vi "ma_Process DC for 1 Block.vi"(6 "reset":bool, 7 "window for DC":T2(ring)=enum."Hanning", 8 "time signal data (samples)":dbl[](array[numeric])=[1.0, 1.0] format="%0.2p", 10 "averaging type":enum16{"Linear", "Exponential"}(ring), 11 "state info":T1 {"buffer" format="%0.2f"; "timestamp" format="%<%.4X>T"; "dt history" format="%0.2f"; "t0 history" format="%<%I:%M:%S%4u %p>T"; "exp TC (samples)" format="%0.2f"; "RMS history" format="%0.2f"; "DC history" format="%0.2f"}) -> (2 "DC value data":dbl=-262128.0 format="%0.6p", 3 "state info":T1 {"buffer" format="%0.2f"; "timestamp" format="%<%.4X>T"; "dt history" format="%0.2f"; "t0 history" format="%<%I:%M:%S%4u %p>T"; "exp TC (samples)" format="%0.2f"; "RMS history" format="%0.2f"; "DC history" format="%0.2f"})   [LabVIEW 2020, in "NI_MAPro.lvlib"]
uses:
  NI_MAPro.lvlib
  NI_AALBase.lvlib
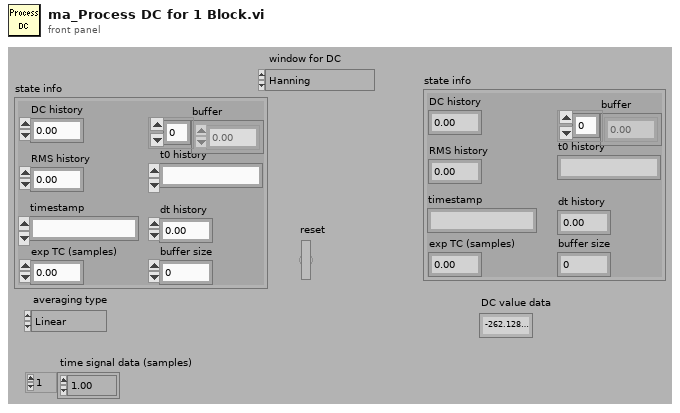
[diagram p1: front panel]
types:
  T1 = cluster{"DC history":dbl, "RMS history":dbl, "exp TC (samples)":dbl, "buffer size":i32, "t0 history":timestamp, "dt history":dbl, "timestamp":timestamp, "buffer":dbl[]}
  T2 = enum16{"Rectangular (none)", "Hanning", "Low side lobe"}
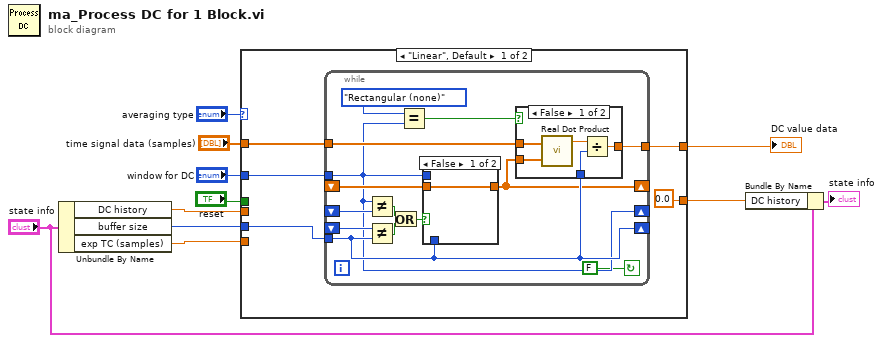
[diagram p0: block diagram]
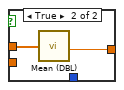
[diagram p2: hidden frame]
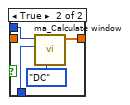
[diagram p3: hidden frame]
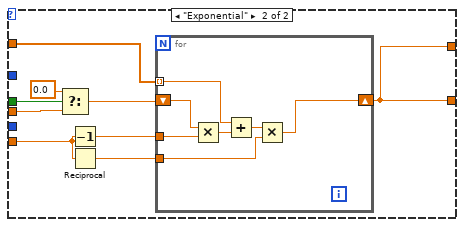
[diagram p4: hidden frame]
diagram:
  n1 = Unbundle By Name("state info") -> ("DC history"=w8:dbl, "buffer size"=w5:i32, "exp TC (samples)"=w7:dbl)
  n2 = case shown="\"Linear\", Default" "averaging type" {
    tunnel: w5 -> [w15 _]
    tunnel: "time signal data (samples)" -> [w14 w51]
    tunnel: [w16 w47] -> w6
    tunnel: w7 -> [_ w49]
    tunnel: [0.0 w47] -> w2
    tunnel: "window for DC" -> [w12 _]
    tunnel: "reset" -> [_ w45]
    tunnel: w8 -> [_ w44]
    frame "Linear", Default {
      n3 = while {
        tunnel: w12 -> [w18]
        shift-left: _ -> [w24]
        shift-right: [w27] -> _
        shift-left: _ -> [w25]
        shift-right: [w28] -> _
        shift-left: _ -> [w26]
        shift-right: [w18] -> _
        tunnel: w14 -> [w29]
        tunnel: w15 -> [w28]
        tunnel: [w30] -> w16
        stop <- FALSE continue-if-true
        n4 = Not Equal?(x=w18, y=w26) -> (x != y?=w23:bool)
        n5 = Not Equal?(x=w25, y=w28) -> (x != y?=w22:bool)
        n6 = Or(x=w23, y=w22) -> (x .or. y?=w21:bool)
        n7 = Equal?(x=T2."Rectangular (none)", y=w18) -> (x = y?=w19:bool)
        n8 = case shown="False" w21 {
          tunnel: w18 -> [_ w42]
          tunnel: w28 -> [_ w41]
          tunnel: [w38 w39] -> w27
          tunnel: w24 -> [w38 _]
          frame False {
          }
          frame True {
            n9 = call "ma_Calculate window.vi"("scaled for"=enum16{"DC", "RMS"}."DC", "array size"=w41, "window"=w42) -> ("Window data"=w39:dbl[])  [unwired: 8 in]
          }
        }
        n10 = case shown="False" w19 {
          tunnel: w29 -> [w35 w37]
          tunnel: [w34 w36] -> w30
          tunnel: w27 -> [w33 _]
          tunnel: w28 -> [w32 _]
          frame False {
            n11 = call "Real Dot Product.vi"("Y Vector"=w33, "X Vector"=w35) -> ("X * Y"=w31:dbl)  [unwired: 1 out]
            n12 = Divide(x=w31, y=w32) -> (x/y=w34:dbl)
          }
          frame True {
            n13 = call "Mean (DBL).vi"("X"=w37) -> ("mean"=w36:dbl)  [unwired: 1 out]
          }
        }
      }
    }
    frame "Exponential" {
      n14 = Select(t=0.0, s=w45, f=w44) -> (s? t:f=w46:dbl)
      n15 = Decrement(x=w49) -> (x-1=w50:dbl)
      n16 = Reciprocal(x=w49) -> (1/x=w48:dbl)
      n17 = for {
        tunnel: w51 -> [w53] mode=indexing
        shift-right: [w52] -> w47
        shift-left: w46 -> [w57]
        tunnel: w50 -> [w58]
        tunnel: w48 -> [w54]
        n18 = Multiply(x=w57, y=w58) -> (x*y=w56:dbl)
        n19 = Add(x=w53, y=w56) -> (x+y=w55:dbl)
        n20 = Multiply(x=w55, y=w54) -> (x*y=w52:dbl)
      }
    }
  }
  "DC value data" <- w6
  n21 = Bundle By Name(cluster="state info", "DC history"=w2) -> (→"state info":T1)
